vi "20170329-bubble_sort_example.vi"() -> ()   [LabVIEW 2014]
panel:
  in  "How many\nnumbers":i32=1024
  out "Origin data":i32[](graph)
  out "Bubble Sort":i32[](graph)
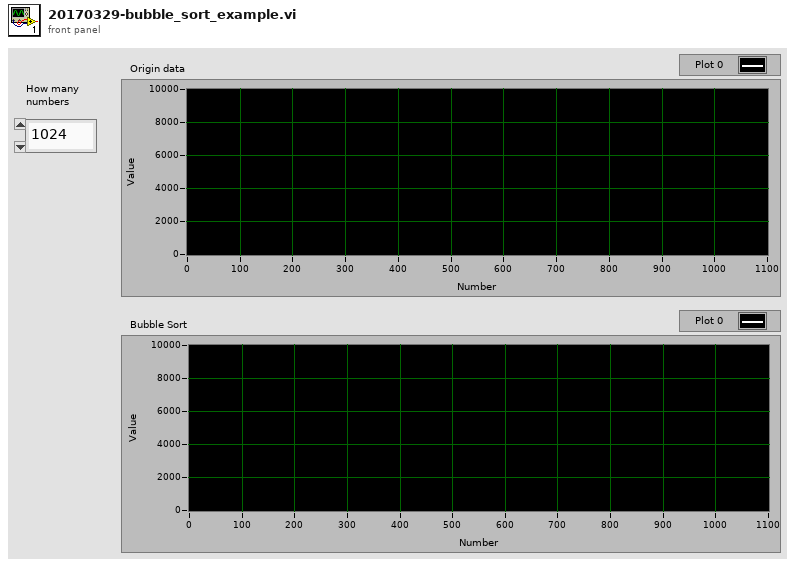
[diagram p1: front panel]
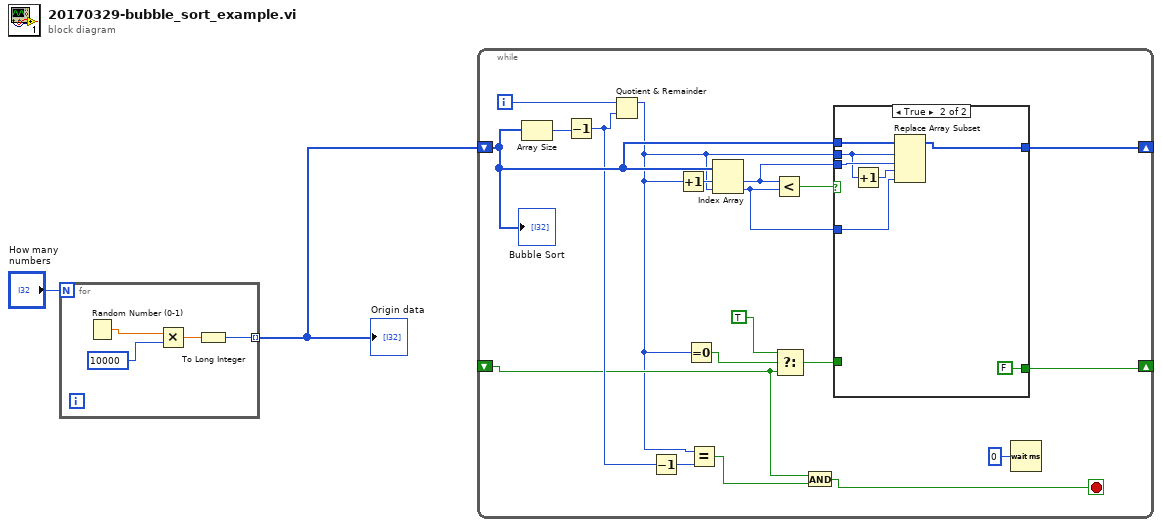
[diagram p0: block diagram]
diagram:
  n1 = for {
    N: "How many\nnumbers" -> [_]
    tunnel: [w3] -> w1 mode=indexing
    n2 = Random Number (0-1)() -> (number: 0 to 1=w6:dbl)
    n3 = Multiply(x=w6, y=10000) -> (x*y=w4:dbl)
    n4 = To Long Integer(number=w4) -> (32bit integer=w3:i32)
  }
  "Origin data" <- w1
  n5 = while {
    shift-right: [w20] -> _
    shift-left: w1 -> [w22]
    shift-right: [w16] -> _
    shift-left: _ -> [w12]
    i -> [w19]
    stop <- w10 stop-if-true
    n6 = Array Size(array=w22) -> (size(s)=w25:i32)
    n7 = Decrement(x=w25) -> (x-1=w13:i32)
    n8 = Quotient & Remainder(x=w19, y=w13) -> (x-y*floor(x/y)=w8:i32)  [unwired: 1 out]
    n9 = Decrement(x=w13) -> (x-1=w14:i32)
    n10 = Increment(x=w8) -> (x+1=w24:i32)
    n11 = Equal To 0?(x=w8) -> (x = 0?=w15:bool)
    n12 = Equal?(x=w8, y=w14) -> (x = y?=w11:bool)
    n13 = Index Array(array=w22, index #1=w24, index #2=w8) -> (element #1=w21:i32, element #2=w9:i32)
    n14 = Less?(x=w21, y=w9) -> (x < y?=w23:bool)
    n15 = Select(t=TRUE, s=w15, f=w12) -> (s? t:f=w17:bool)
    n16 = And(x=w12, y=w11) -> (x .and. y?=w10:bool)
    n17 = case shown="True" w23 {
      tunnel: w8 -> [_ w30]
      tunnel: w22 -> [w27 w34]
      tunnel: w21 -> [_ w33]
      tunnel: w9 -> [_ w32]
      tunnel: [w27 w29] -> w20
      tunnel: w17 -> [w26 _]
      tunnel: [w26 FALSE] -> w16
      frame False {
      }
      frame True {
        n18 = Increment(x=w30) -> (x+1=w31:i32)
        n19 = Replace Array Subset(array=w34, new element #1=w33, index #1=w30, new element #2=w32, index #2=w31) -> (w29:i32[])
      }
    }
    n20 = Wait (ms)(milliseconds to wait=u32 0) -> ()  [unwired: 1 out]
    "Bubble Sort" <- w22
  }
